vi "Pneumatic_Open.vi"   [LabVIEW 2016]
uses:
  <vilib>/Rock Robotics/WPI/Utilities/WPI_GetSetVariantRefNum.vi
types:
  T1 = typedef "WPI_CompressorDevRef.ctl" = cluster{"DevStatus":errorcluster, "Pneumatics Control Module":u8}
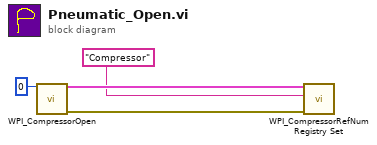
[diagram p0: block diagram]
diagram:
  n1 = call <vilib>:"WPI_CompressorOpen.vi"("Pneumatics Control Module (0)"=u8 0) -> ("CompressorDevRef"=w3:T1, "error out"=w4:errorcluster)  [unwired: 13 in]
  n2 = call <vilib>:"WPI_CompressorRefNum Registry Set.vi"("error in (no error)"=w4, "refnum name"="Compressor", "CompressorDevRef"=w3) -> ()  [unwired: 7 in, 2 out]
